vi "Utility_OpenVI FP and Bring it to Front.vi"(8 "error in (no error)":errorcluster, 11 "VI Path":path) -> (0 "error out":errorcluster)   [LabVIEW 2024]
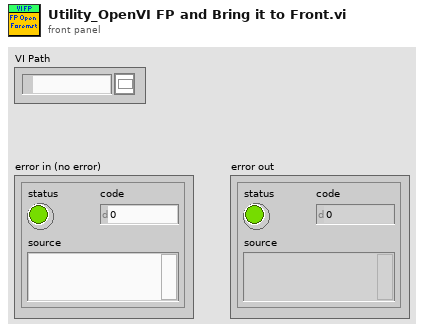
[diagram p1: front panel]
types:
  T1 = enum32{"Invalid", "Standard", "Closed", "Hidden", "Minimized", "Maximized"}
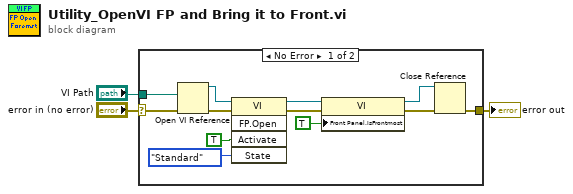
[diagram p0: block diagram]
diagram:
  n1 = case shown="No Error" "error in (no error)" {
    selector: "error in (no error)" -> [w4 w16]
    tunnel: "VI Path" -> [w15 _]
    tunnel: [w6 w16] -> w2
    frame No Error {
      n2 = Open VI Reference(vi path=w15, error in (no error)=w4) -> (vi reference=w14:refnum<vi>, error out=w11:errorcluster)  [unwired: 4 in]
      n3 = invoke class="VI" method="FP.Open"(reference=w14, error in=w11, "Activate"=TRUE ("Activate?"), "State"=T1."Standard") -> (reference out=w9:refnum<vi>, error out=w10:errorcluster)  [unwired: 1 in, 3 out]
      n4 = property class="VI"(reference=w9, error in=w10, "Front Panel.IsFrontmost"=TRUE ("Front Panel Window:Is Frontmost")) -> (reference out=w5:refnum<vi>, error out=w7:errorcluster)
      n5 = Close Reference(reference=w5, error in (no error)=w7) -> (error out=w6:errorcluster)
    }
    frame Error {
    }
  }
  "error out" <- w2
